vi "Get_nmr DATA.vi"(11 "file path (dialog if empty)":path=path "E:/PHD/uwave/Microwave_VI_V3/Pol_Out.csv") -> (3 "Last Row":string[](array[string]))   [LabVIEW 2019]
uses:
  <vilib>/Utility/file.llb/Read Delimited Spreadsheet (string).vi
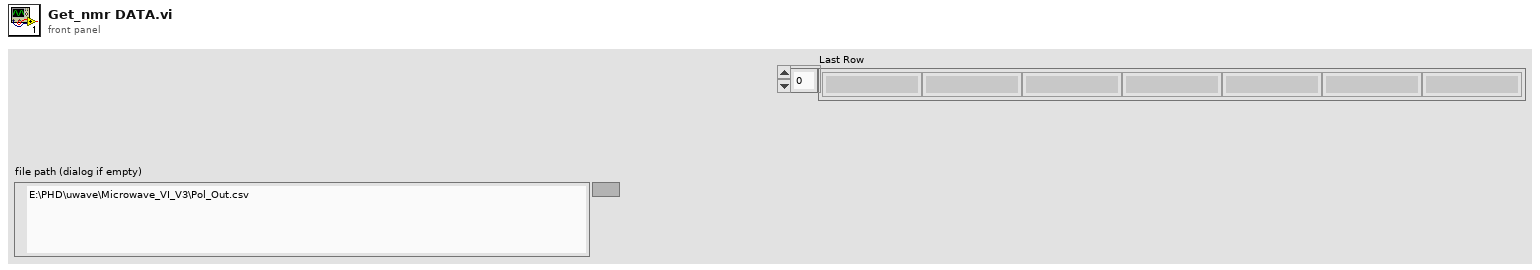
[diagram p1: front panel]
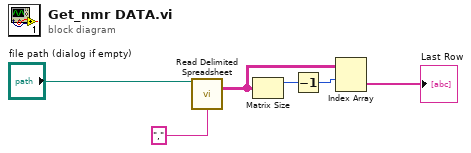
[diagram p0: block diagram]
diagram:
  n1 = call-poly <vilib>:"Read Delimited Spreadsheet.vi"("file path (dialog if empty)"="file path (dialog if empty)", "delimiter (\\t)"="," ("delimiter (\\t)")) -> ("all rows"=w4:string[][])  [unwired: 8 in, 5 out]
  n2 = Matrix Size(0:w4) -> (1:w2:i32)  [unwired: 1 out]
  n3 = Decrement(x=w2) -> (x-1=w3:i32)
  n4 = Index Array(array=w4, index (row)=w3) -> (element=→"Last Row":string[])  [unwired: 1 in]
